vi "Flatten.vi"(8 "error in":errorcluster, 10 "Data":T1) -> (0 "error out":errorcluster, 2 "Buffer":u8[](array[numeric]) format="%.0x")   [LabVIEW 2020, in "PB Msg Template.lvlib"]
uses:
  PB Msg Template.lvlib
  Data.ctl
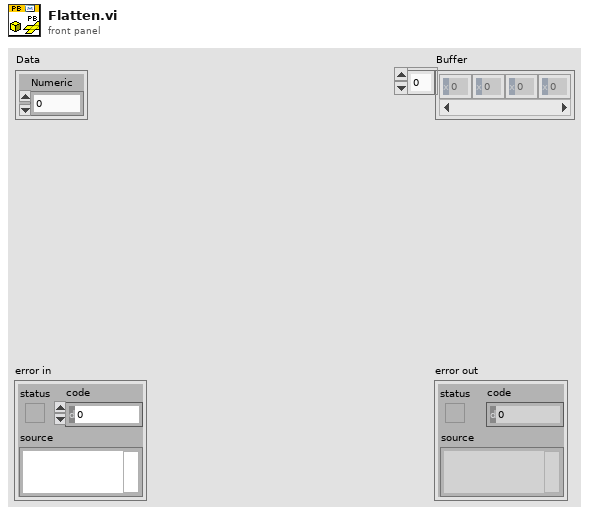
[diagram p1: front panel]
types:
  T1 = typedef "PB Msg Template.lvlib/Data.ctl" = cluster{"Numeric":dbl}
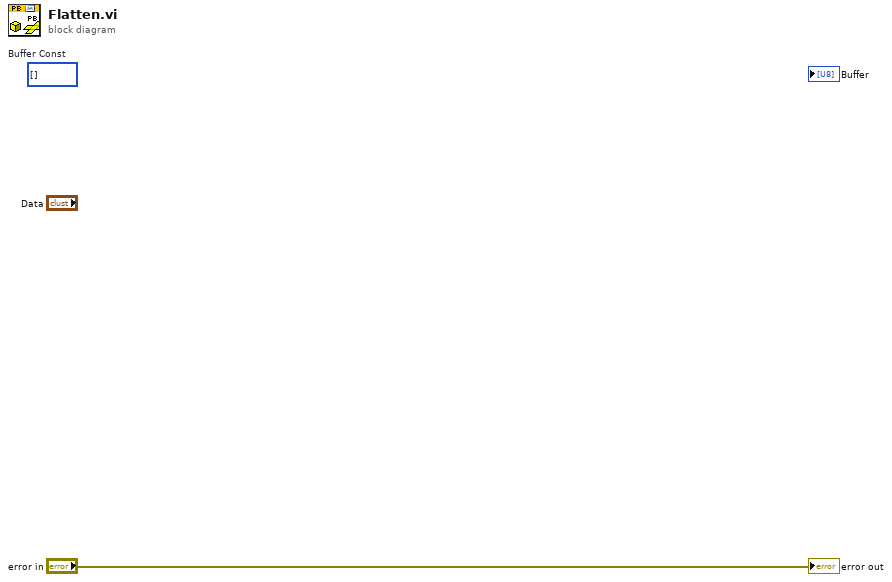
[diagram p0: block diagram]
diagram:
  (unwired) u8[] []  # Buffer Const
  "error out" <- "error in"
